vi "Constant - Default Port Number.vi"() -> (3 "Port":u16=9760)   [LabVIEW 2020]
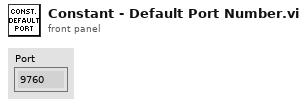
[diagram p1: front panel]
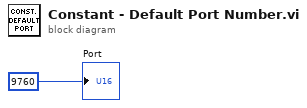
[diagram p0: block diagram]
diagram:
  "Port" <- u16 9760 ("remote port or service name")
